vi "to posint fixint.vi"(8 "error in":errorcluster, 11 "byte in":u8) -> (0 "error out":errorcluster, 3 "posint":u8)   [LabVIEW 2020, in "wamplv.lvlib" / "MessagePack.lvclass"]
uses:
  MessagePack.lvclass
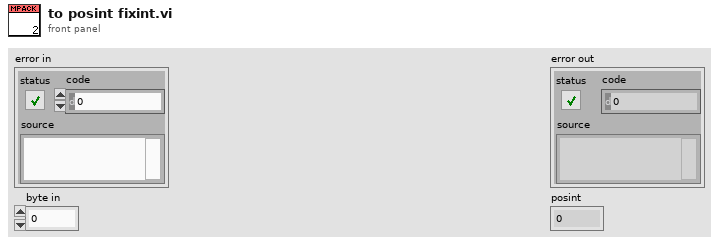
[diagram p1: front panel]
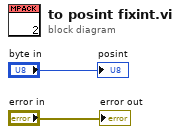
[diagram p0: block diagram]
diagram:
  "error out" <- "error in"
  "posint" <- "byte in"
